vi "HiPace1200_Test.vi"() -> ()   [LabVIEW 2019]
panel:
  in  "CtrlViaInt_in":u8=255
  in  "get_motor_onoff":bool
  out "motor_onoff":string
  out "pump_st_onoff":string
  in  "get_pump_st_onoff":bool
  in  "set_IntSelLckd":bool
  out "IntSelLckd_out":string
  out "IntSelLckd":string
  in  "get_IntSelLckd":bool
  in  "set_CtrlViaInt":bool
  out "ctrl_via_int_out":i16
  in  "get_CtrlViaInt":bool
  out "ctrl_via_int":i16
  in  "reconnect":bool
  in  "ack_error_1":bool
  out "ack_error_1_ret":string
  in  "get_elec_name":bool
  out "elec_name":string
  in  "get_gas_flow":bool
  out "gas_flow":i16 caption="sccm"
  in  "get_accel":bool
  out "accel":i16 caption="rpm/s"
  in  "get_temp_rotor":bool
  out "temp_rotor":i16 caption="degC"
  in  "get_temp_motor":bool
  out "temp_motor":i16 caption="degC"
  in  "get_temp_bearng":bool
  out "temp_bearng":i16 caption="degC"
  in  "get_temp_pmp_bot":bool
  out "temp_pmp_bot":i16 caption="degC"
  in  "get_temp_elec":bool
  out "temp_elec":i16 caption="degC"
  in  "get_rot_spd_nom":bool
  out "rot_speed_nom":i16 caption="Hz"
  in  "get_temp_pwr_stg":bool
  out "temp_pwr_stg":i16 caption="degC"
  in  "get_rot_spd_s":bool
  out "rot_speed_sp":i16 caption="Hz"
  out "rot_speed_r":i16 caption="Hz"
  in  "get_rot_spd_r":bool
  in  "ack_error":bool
  out "ack_error_ret":string
  out "error_code":string
  in  "get_error_code":bool
  in  "turn_off_motor":bool
  in  "turn_on_motor":bool
  in  "turn_off_pump_st":bool
  in  "turn_on_pump_st":bool
  in  "device_addr":u16=1
  out "raw_response":string
  in  "port":u16=4196
  in  "ip_addr":string="192.168.24.133"
  out "time":timestamp format="%<%Y-%m-%d %H:%M:%S>T"
  out "status":bool
  in  "timeout":u32=1000
  in  "stop":bool
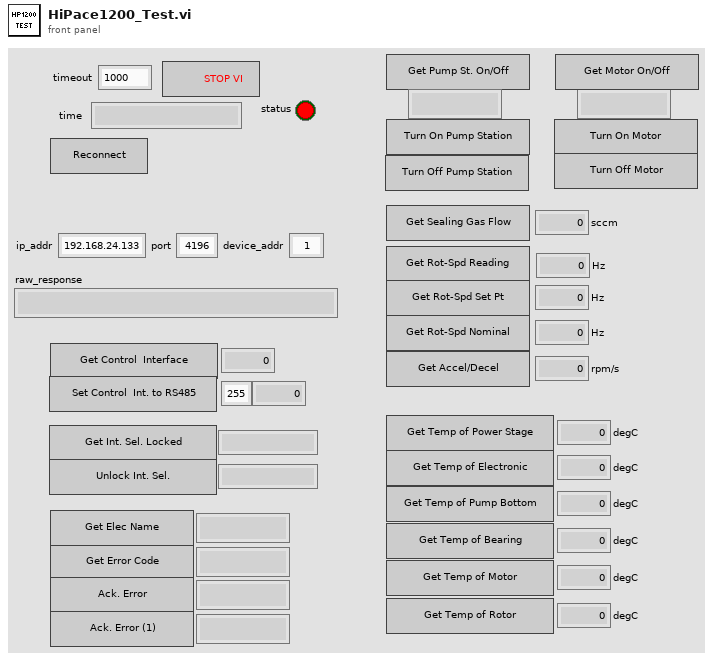
[diagram p1: front panel]
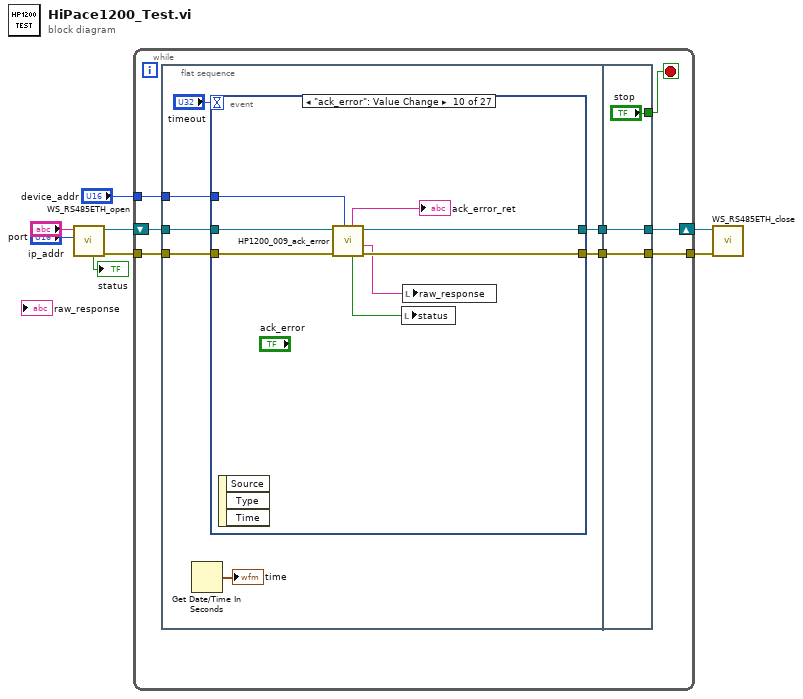
[diagram p0: block diagram]
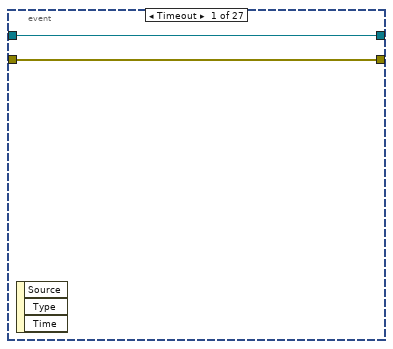
[diagram p2: hidden frame]
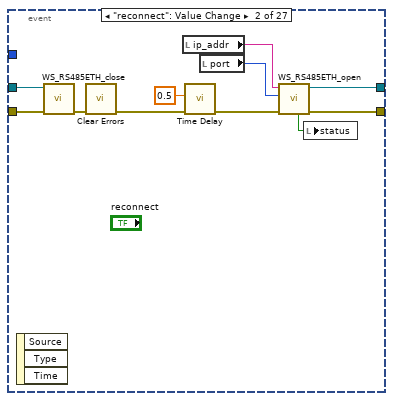
[diagram p3: hidden frame]
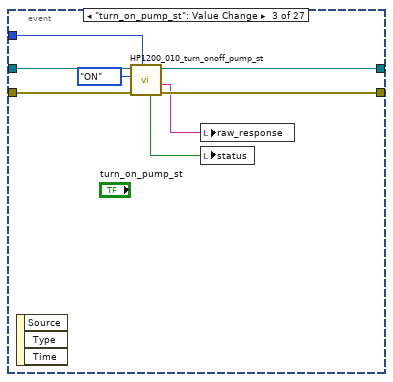
[diagram p4: hidden frame]
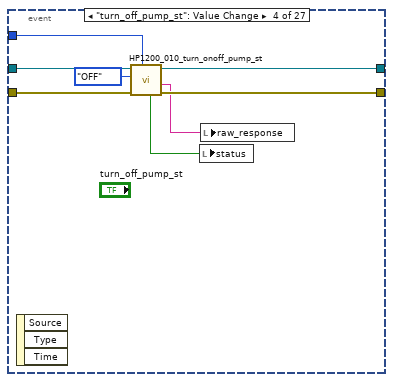
[diagram p5: hidden frame]
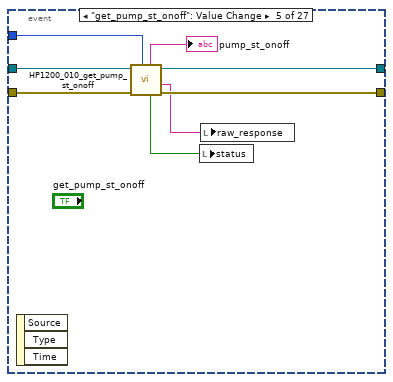
[diagram p6: hidden frame]
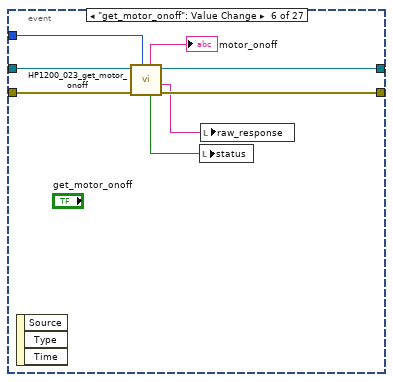
[diagram p7: hidden frame]
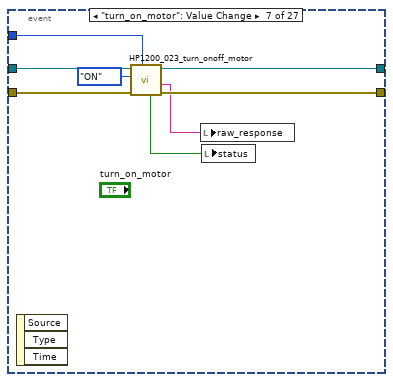
[diagram p8: hidden frame]
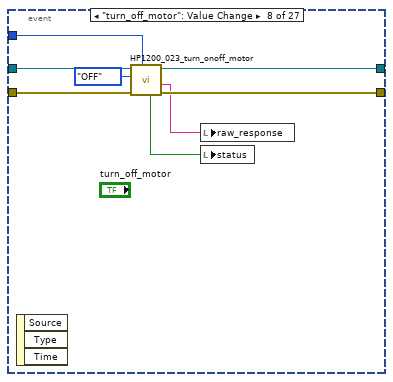
[diagram p9: hidden frame]
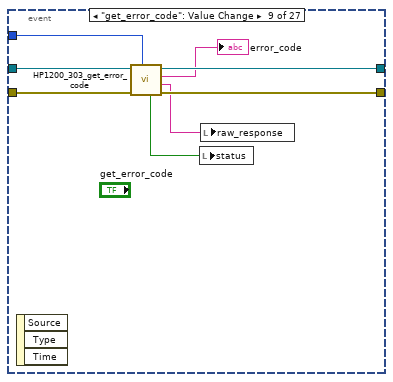
[diagram p10: hidden frame]
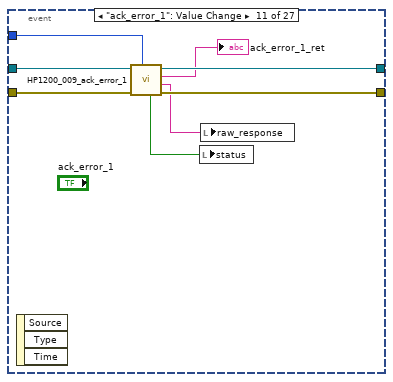
[diagram p11: hidden frame]
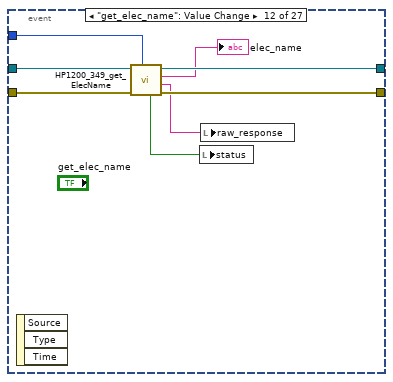
[diagram p12: hidden frame]
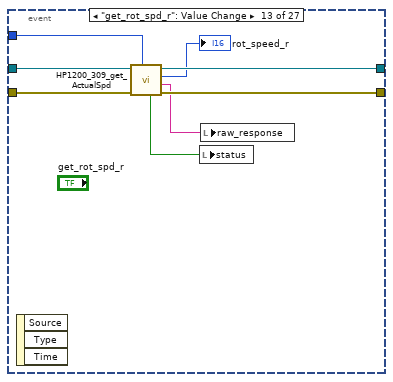
[diagram p13: hidden frame]
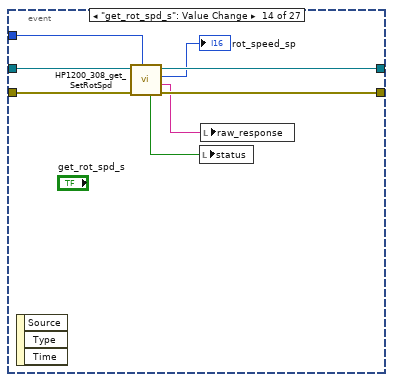
[diagram p14: hidden frame]
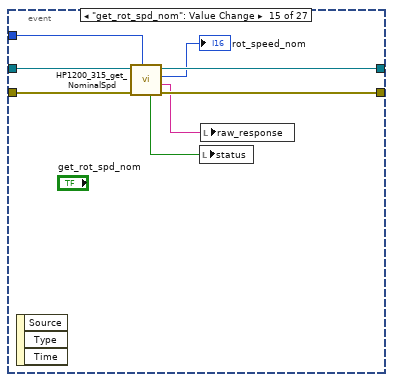
[diagram p15: hidden frame]
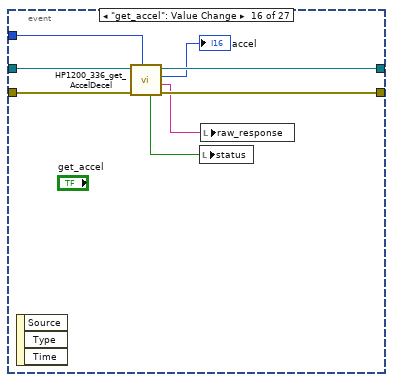
[diagram p16: hidden frame]
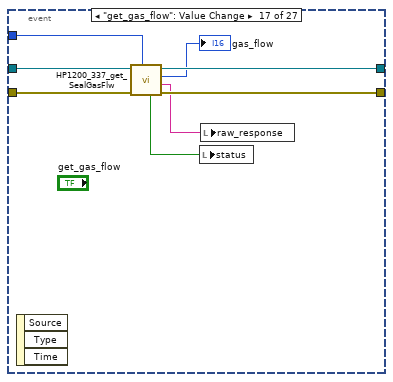
[diagram p17: hidden frame]
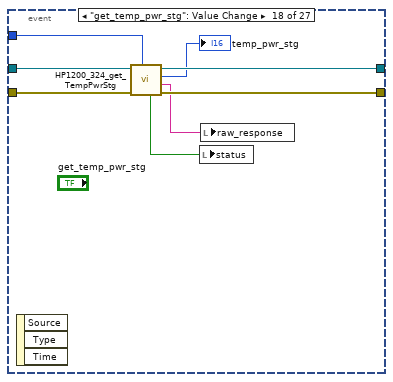
[diagram p18: hidden frame]
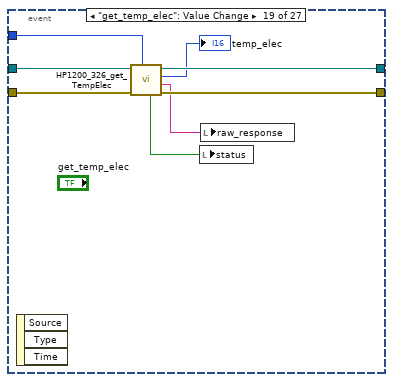
[diagram p19: hidden frame]
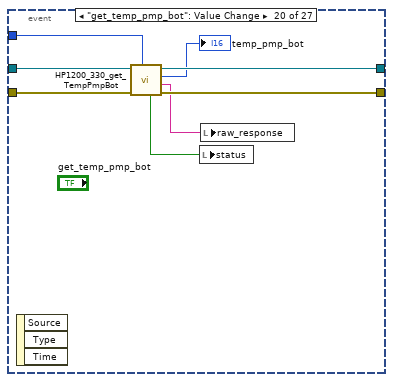
[diagram p20: hidden frame]
diagram:
  n1 = call "WS_RS485ETH_open.vi"("port"="port", "ip_addr"="ip_addr") -> ("error out"=w6:errorcluster, "conn_id"=w8:refnum<k5>, "status"=→"status":bool)  [unwired: 7 in]
  n2 = while {
    tunnel: w6 -> [w12]
    tunnel: [w10] -> w5
    tunnel: "device_addr" -> [w9]
    shift-right: [w13] -> w7
    shift-left: w8 -> [w15]
    stop <- w16 stop-if-true
    n3 = flat-sequence {
      tunnel: w15 -> [w23]
      tunnel: [w22] -> w14
      tunnel: w12 -> [w21]
      tunnel: [w20] -> w11
      tunnel: w9 -> [w18]
      tunnel: ["stop"] -> w16
      tunnel: w14 -> [w240]
      tunnel: [w240] -> w13
      tunnel: w11 -> [w239]
      tunnel: [w239] -> w10
      frame #0 {
        n4 = Get Date/Time In Seconds() -> (seconds since 1Jan1904=→"time":timestamp)
        n5 = event shown="[9] \"ack_error\": Value Change" {
          selector: _ -> [_ _ _ _ _ _ _ _ _ _ _ _ _ _ _ _ _ _ _ _ _ _ _ _ _ _ _]
          dyn-events: _ -> [_ _ _ _ _ _ _ _ _ _ _ _ _ _ _ _ _ _ _ _ _ _ _ _ _ _ _]
          timeout: "timeout" -> [_ _ _ _ _ _ _ _ _ _ _ _ _ _ _ _ _ _ _ _ _ _ _ _ _ _ _]
          tunnel: w23 -> [w25 w36 w44 w52 w60 w68 w76 w84 w92 w100 w108 w116 w124 w132 w140 w148 w156 w164 w172 w180 w188 w196 w204 w212 w221 w229 w238]
          tunnel: [w25 w34 w42 w50 w58 w66 w74 w82 w90 w98 w106 w114 w122 w130 w138 w146 w154 w162 w170 w178 w186 w194 w202 w210 w219 w227 w236] -> w22
          tunnel: w21 -> [w24 w35 w43 w51 w59 w67 w75 w83 w91 w99 w107 w115 w123 w131 w139 w147 w155 w163 w171 w179 w187 w195 w203 w211 w220 w228 w237]
          tunnel: [w24 w33 w41 w49 w57 w65 w73 w81 w89 w97 w105 w113 w121 w129 w137 w145 w153 w161 w169 w177 w185 w193 w201 w209 w218 w226 w235] -> w20
          tunnel: w18 -> [_ _ w40 w48 w56 w64 w72 w80 w88 w96 w104 w112 w120 w128 w136 w144 w152 w160 w168 w176 w184 w192 w200 w208 w217 w225 w234]
          event Timeout {
            n6 = event-data() -> ()  [unwired: 1 in, 3 out]
          }
          event "reconnect": Value Change {
            n7 = event-data() -> ()  [unwired: 1 in, 3 out]
            n8 = call "WS_RS485ETH_close.vi"("error in"=w35, "conn_id"=w36) -> ("error out"=w30:errorcluster)  [unwired: 8 in, 1 out]
            n9 = call <vilib>:"Clear Errors.vi"("error in (no error)"=w30) -> ("error out"=w28:errorcluster)  [unwired: 5 in, 1 out]
            n10 = local read "ip_addr"() -> (w31:string)
            n11 = call "Time Delay"("error in (no error)"=w28, "Delay Time (s)"=0.5) -> ("error out"=w27:errorcluster)  [unwired: 9 in]
            n12 = local read "port"() -> (w32:u16)
            n13 = call "WS_RS485ETH_open.vi"("error in"=w27, "port"=w32, "ip_addr"=w31) -> ("error out"=w33:errorcluster, "conn_id"=w34:refnum<k5>, "status"=w29:bool)  [unwired: 6 in]
            n14 = local write "status"(w29) -> ()
          }
          event "turn_on_pump_st": Value Change {
            n15 = event-data() -> ()  [unwired: 1 in, 3 out]
            n16 = call "HP1200_010_turn_onoff_pump_st.vi"("device_addr"=w40, "error in"=w43, "onoff"=enum16{"ON", "OFF"}."ON", "conn_id_in"=w44) -> ("error out"=w41:errorcluster, "response"=w38:string, "conn_id_out"=w42:refnum<k5>, "status"=w37:bool)  [unwired: 3 in, 1 out]
            n17 = local write "raw_response"(w38) -> ()
            n18 = local write "status"(w37) -> ()
          }
          event "turn_off_pump_st": Value Change {
            n19 = event-data() -> ()  [unwired: 1 in, 3 out]
            n20 = call "HP1200_010_turn_onoff_pump_st.vi"("device_addr"=w48, "error in"=w51, "onoff"=enum16{"ON", "OFF"}."OFF", "conn_id_in"=w52) -> ("error out"=w49:errorcluster, "response"=w46:string, "conn_id_out"=w50:refnum<k5>, "status"=w45:bool)  [unwired: 3 in, 1 out]
            n21 = local write "status"(w45) -> ()
            n22 = local write "raw_response"(w46) -> ()
          }
          event "get_pump_st_onoff": Value Change {
            n23 = event-data() -> ()  [unwired: 1 in, 3 out]
            n24 = call "HP1200_010_get_pump_st_onoff.vi"("device_addr"=w56, "error in"=w59, "conn_id_in"=w60) -> ("error out"=w57:errorcluster, "response"=w55:string, "conn_id_out"=w58:refnum<k5>, "status"=w54:bool, "onoff_ret"=→"pump_st_onoff":string)  [unwired: 3 in, 1 out]
            n25 = local write "status"(w54) -> ()
            n26 = local write "raw_response"(w55) -> ()
          }
          event "get_motor_onoff": Value Change {
            n27 = event-data() -> ()  [unwired: 1 in, 3 out]
            n28 = call "HP1200_023_get_motor_onoff.vi"("device_addr"=w64, "error in"=w67, "conn_id_in"=w68) -> ("error out"=w65:errorcluster, "response"=w63:string, "conn_id_out"=w66:refnum<k5>, "status"=w62:bool, "onoff_ret"=→"motor_onoff":string)  [unwired: 3 in, 1 out]
            n29 = local write "status"(w62) -> ()
            n30 = local write "raw_response"(w63) -> ()
          }
          event "turn_on_motor": Value Change {
            n31 = event-data() -> ()  [unwired: 1 in, 3 out]
            n32 = call "HP1200_023_turn_onoff_motor.vi"("device_addr"=w72, "error in"=w75, "onoff"=enum16{"ON", "OFF"}."ON", "conn_id_in"=w76) -> ("error out"=w73:errorcluster, "response"=w70:string, "conn_id_out"=w74:refnum<k5>, "status"=w69:bool)  [unwired: 3 in, 1 out]
            n33 = local write "raw_response"(w70) -> ()
            n34 = local write "status"(w69) -> ()
          }
          event "turn_off_motor": Value Change {
            n35 = event-data() -> ()  [unwired: 1 in, 3 out]
            n36 = call "HP1200_023_turn_onoff_motor.vi"("device_addr"=w80, "error in"=w83, "onoff"=enum16{"ON", "OFF"}."OFF", "conn_id_in"=w84) -> ("error out"=w81:errorcluster, "response"=w78:string, "conn_id_out"=w82:refnum<k5>, "status"=w77:bool)  [unwired: 3 in, 1 out]
            n37 = local write "raw_response"(w78) -> ()
            n38 = local write "status"(w77) -> ()
          }
          event "get_error_code": Value Change {
            n39 = event-data() -> ()  [unwired: 1 in, 3 out]
            n40 = call "HP1200_303_get_error_code.vi"("device_addr"=w88, "error in"=w91, "conn_id_in"=w92) -> ("error out"=w89:errorcluster, "response"=w87:string, "error_code"=→"error_code":string, "conn_id_out"=w90:refnum<k5>, "status"=w85:bool)  [unwired: 4 in]
            n41 = local write "status"(w85) -> ()
            n42 = local write "raw_response"(w87) -> ()
          }
          event "ack_error": Value Change {
            n43 = event-data() -> ()  [unwired: 1 in, 3 out]
            n44 = call "HP1200_009_ack_error.vi"("device_addr"=w96, "error in"=w99, "conn_id_in"=w100) -> ("error out"=w97:errorcluster, "response"=w95:string, "conn_id_out"=w98:refnum<k5>, "status"=w94:bool, "ack_ret"=→"ack_error_ret":string)  [unwired: 3 in, 1 out]
            n45 = local write "status"(w94) -> ()
            n46 = local write "raw_response"(w95) -> ()
          }
          event "ack_error_1": Value Change {
            n47 = event-data() -> ()  [unwired: 1 in, 3 out]
            n48 = call "HP1200_009_ack_error_1.vi"("device_addr"=w104, "error in"=w107, "conn_id_in"=w108) -> ("error out"=w105:errorcluster, "response"=w103:string, "ack_ret"=→"ack_error_1_ret":string, "conn_id_out"=w106:refnum<k5>, "status"=w101:bool)  [unwired: 4 in]
            n49 = local write "status"(w101) -> ()
            n50 = local write "raw_response"(w103) -> ()
          }
          event "get_elec_name": Value Change {
            n51 = event-data() -> ()  [unwired: 1 in, 3 out]
            n52 = call "HP1200_349_get_ElecName.vi"("device_addr"=w112, "error in"=w115, "conn_id_in"=w116) -> ("error out"=w113:errorcluster, "response"=w111:string, "elec_name"=→"elec_name":string, "conn_id_out"=w114:refnum<k5>, "status"=w109:bool)  [unwired: 4 in]
            n53 = local write "status"(w109) -> ()
            n54 = local write "raw_response"(w111) -> ()
          }
          event "get_rot_spd_r": Value Change {
            n55 = event-data() -> ()  [unwired: 1 in, 3 out]
            n56 = call "HP1200_309_get_ActualSpd.vi"("device_addr"=w120, "error in"=w123, "conn_id_in"=w124) -> ("error out"=w121:errorcluster, "response"=w119:string, "rot_speed"=→"rot_speed_r":i16, "conn_id_out"=w122:refnum<k5>, "status"=w118:bool)  [unwired: 4 in]
            n57 = local write "status"(w118) -> ()
            n58 = local write "raw_response"(w119) -> ()
          }
          event "get_rot_spd_s": Value Change {
            n59 = event-data() -> ()  [unwired: 1 in, 3 out]
            n60 = call "HP1200_308_get_SetRotSpd.vi"("device_addr"=w128, "error in"=w131, "conn_id_in"=w132) -> ("error out"=w129:errorcluster, "response"=w127:string, "rot_speed"=→"rot_speed_sp":i16, "conn_id_out"=w130:refnum<k5>, "status"=w126:bool)  [unwired: 4 in]
            n61 = local write "status"(w126) -> ()
            n62 = local write "raw_response"(w127) -> ()
          }
          event "get_rot_spd_nom": Value Change {
            n63 = event-data() -> ()  [unwired: 1 in, 3 out]
            n64 = call "HP1200_315_get_NominalSpd.vi"("device_addr"=w136, "error in"=w139, "conn_id_in"=w140) -> ("error out"=w137:errorcluster, "response"=w135:string, "rot_speed"=→"rot_speed_nom":i16, "conn_id_out"=w138:refnum<k5>, "status"=w134:bool)  [unwired: 4 in]
            n65 = local write "status"(w134) -> ()
            n66 = local write "raw_response"(w135) -> ()
          }
          event "get_accel": Value Change {
            n67 = event-data() -> ()  [unwired: 1 in, 3 out]
            n68 = call "HP1200_336_get_AccelDecel.vi"("device_addr"=w144, "error in"=w147, "conn_id_in"=w148) -> ("error out"=w145:errorcluster, "response"=w143:string, "acc"=→"accel":i16, "conn_id_out"=w146:refnum<k5>, "status"=w142:bool)  [unwired: 4 in]
            n69 = local write "status"(w142) -> ()
            n70 = local write "raw_response"(w143) -> ()
          }
          event "get_gas_flow": Value Change {
            n71 = event-data() -> ()  [unwired: 1 in, 3 out]
            n72 = call "HP1200_337_get_SealGasFlw.vi"("device_addr"=w152, "error in"=w155, "conn_id_in"=w156) -> ("error out"=w153:errorcluster, "response"=w151:string, "flow"=→"gas_flow":i16, "conn_id_out"=w154:refnum<k5>, "status"=w150:bool)  [unwired: 4 in]
            n73 = local write "status"(w150) -> ()
            n74 = local write "raw_response"(w151) -> ()
          }
          event "get_temp_pwr_stg": Value Change {
            n75 = event-data() -> ()  [unwired: 1 in, 3 out]
            n76 = call "HP1200_324_get_TempPwrStg.vi"("device_addr"=w160, "error in"=w163, "conn_id_in"=w164) -> ("error out"=w161:errorcluster, "response"=w159:string, "temp"=→"temp_pwr_stg":i16, "conn_id_out"=w162:refnum<k5>, "status"=w158:bool)  [unwired: 4 in]
            n77 = local write "status"(w158) -> ()
            n78 = local write "raw_response"(w159) -> ()
          }
          event "get_temp_elec": Value Change {
            n79 = event-data() -> ()  [unwired: 1 in, 3 out]
            n80 = call "HP1200_326_get_TempElec.vi"("device_addr"=w168, "error in"=w171, "conn_id_in"=w172) -> ("error out"=w169:errorcluster, "response"=w167:string, "temp"=→"temp_elec":i16, "conn_id_out"=w170:refnum<k5>, "status"=w166:bool)  [unwired: 4 in]
            n81 = local write "status"(w166) -> ()
            n82 = local write "raw_response"(w167) -> ()
          }
          event "get_temp_pmp_bot": Value Change {
            n83 = event-data() -> ()  [unwired: 1 in, 3 out]
            n84 = call "HP1200_330_get_TempPmpBot.vi"("device_addr"=w176, "error in"=w179, "conn_id_in"=w180) -> ("error out"=w177:errorcluster, "response"=w175:string, "temp"=→"temp_pmp_bot":i16, "conn_id_out"=w178:refnum<k5>, "status"=w174:bool)  [unwired: 4 in]
            n85 = local write "status"(w174) -> ()
            n86 = local write "raw_response"(w175) -> ()
          }
          event "get_temp_bearng": Value Change {
            n87 = event-data() -> ()  [unwired: 1 in, 3 out]
            n88 = call "HP1200_342_get_TempBearng.vi"("device_addr"=w184, "error in"=w187, "conn_id_in"=w188) -> ("error out"=w185:errorcluster, "response"=w183:string, "temp"=→"temp_bearng":i16, "conn_id_out"=w186:refnum<k5>, "status"=w182:bool)  [unwired: 4 in]
            n89 = local write "status"(w182) -> ()
            n90 = local write "raw_response"(w183) -> ()
          }
          event "get_temp_motor": Value Change {
            n91 = event-data() -> ()  [unwired: 1 in, 3 out]
            n92 = call "HP1200_346_get_TempMotor.vi"("device_addr"=w192, "error in"=w195, "conn_id_in"=w196) -> ("error out"=w193:errorcluster, "response"=w191:string, "temp"=→"temp_motor":i16, "conn_id_out"=w194:refnum<k5>, "status"=w190:bool)  [unwired: 4 in]
            n93 = local write "status"(w190) -> ()
            n94 = local write "raw_response"(w191) -> ()
          }
          event "get_temp_rotor": Value Change {
            n95 = event-data() -> ()  [unwired: 1 in, 3 out]
            n96 = call "HP1200_384_get_TempRotor.vi"("device_addr"=w200, "error in"=w203, "conn_id_in"=w204) -> ("error out"=w201:errorcluster, "response"=w199:string, "temp"=→"temp_rotor":i16, "conn_id_out"=w202:refnum<k5>, "status"=w198:bool)  [unwired: 4 in]
            n97 = local write "status"(w198) -> ()
            n98 = local write "raw_response"(w199) -> ()
          }
          event "get_CtrlViaInt": Value Change {
            n99 = event-data() -> ()  [unwired: 1 in, 3 out]
            n100 = call "HP1200_060_get_CtrlViaInt.vi"("device_addr"=w208, "error in"=w211, "conn_id_in"=w212) -> ("error out"=w209:errorcluster, "response"=w207:string, "CtrlViaInt"=→"ctrl_via_int":u8, "conn_id_out"=w210:refnum<k5>, "status"=w206:bool)  [unwired: 4 in]
            n101 = local write "status"(w206) -> ()
            n102 = local write "raw_response"(w207) -> ()
          }
          event "set_CtrlViaInt": Value Change {
            n103 = event-data() -> ()  [unwired: 1 in, 3 out]
            n104 = call "HP1200_060_set_CtrlViaInt.vi"("device_addr"=w217, "error in"=w220, "CtrlViaInt_in"="CtrlViaInt_in", "conn_id_in"=w221) -> ("error out"=w218:errorcluster, "response"=w216:string, "CtrlViaInt"=→"ctrl_via_int_out":u8, "conn_id_out"=w219:refnum<k5>, "status"=w215:bool)  [unwired: 3 in]
            n105 = local write "status"(w215) -> ()
            n106 = local write "raw_response"(w216) -> ()
          }
          event "get_IntSelLckd": Value Change {
            n107 = event-data() -> ()  [unwired: 1 in, 3 out]
            n108 = call "HP1200_061_get_IntSelLckd.vi"("device_addr"=w225, "error in"=w228, "conn_id_in"=w229) -> ("error out"=w226:errorcluster, "response"=w224:string, "locked"=→"IntSelLckd":string, "conn_id_out"=w227:refnum<k5>, "status"=w223:bool)  [unwired: 4 in]
            n109 = local write "status"(w223) -> ()
            n110 = local write "raw_response"(w224) -> ()
          }
          event "set_IntSelLckd": Value Change {
            n111 = event-data() -> ()  [unwired: 1 in, 3 out]
            n112 = call "HP1200_061_set_IntSelLckd.vi"("device_addr"=w234, "error in"=w237, "onoff"=enum16{"ON", "OFF"}."OFF", "conn_id_in"=w238) -> ("error out"=w235:errorcluster, "response"=w233:string, "onoff_ret"=→"IntSelLckd_out":string, "conn_id_out"=w236:refnum<k5>, "status"=w232:bool)  [unwired: 3 in]
            n113 = local write "status"(w232) -> ()
            n114 = local write "raw_response"(w233) -> ()
          }
        }
      }
      frame #1 {
      }
    }
  }
  n115 = call "WS_RS485ETH_close.vi"("error in"=w5, "conn_id"=w7) -> ()  [unwired: 8 in, 2 out]
